vi "Read Default Values.vi"(0 "Queue Ref":refnum<queue>, 5 "Empty string?":bool, 11 "error in":errorcluster) -> (15 "error out":errorcluster)   [LabVIEW 2021]
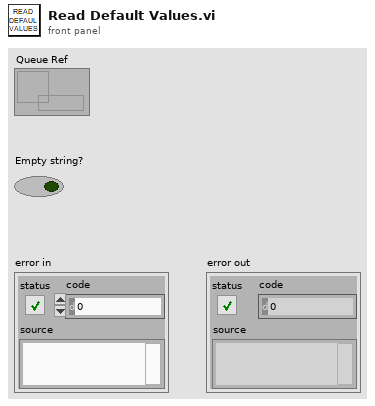
[diagram p1: front panel]
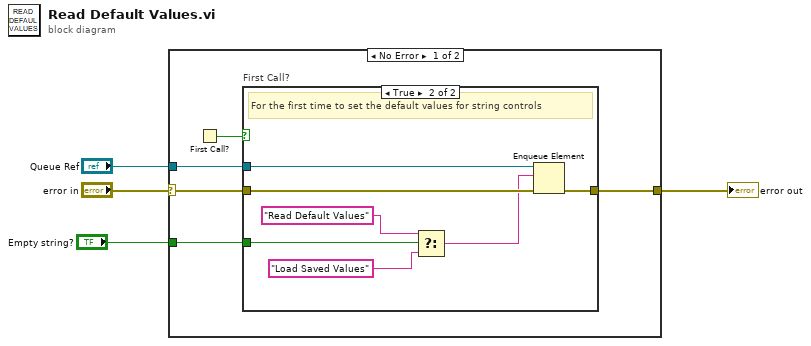
[diagram p0: block diagram]
diagram:
  n1 = case shown="No Error" "error in" {
    selector: "error in" -> [w9 w18]
    tunnel: [w8 w18] -> w3
    tunnel: "Queue Ref" -> [w7 _]
    tunnel: "Empty string?" -> [w5 _]
    frame No Error {
      n2 = First Call?() -> (First Call?: T/F=w6:bool)
      n3 = case "First Call?" shown="True" w6 {
        tunnel: w9 -> [w10 w17]
        tunnel: [w10 w16] -> w8
        tunnel: w7 -> [_ w15]
        tunnel: w5 -> [_ w12]
        frame False {
        }
        frame True {
          # "For the first time to set the default values for string controls"
          n4 = Select(t="Read Default Values" ("element"), s=w12, f="Load Saved Values" ("element")) -> (s? t:f=w11:string)
          n5 = Enqueue Element(queue=w15, element=w11, error in (no error)=w17) -> (error out=w16:errorcluster)  [unwired: 1 in, 2 out]
        }
      }
    }
    frame Error {
    }
  }
  "error out" <- w3
